vi "setCurrent.vi"(8 "error in (no error)":errorcluster, 11 "curent set":u16) -> (0 "error out":errorcluster)   [LabVIEW 2013]
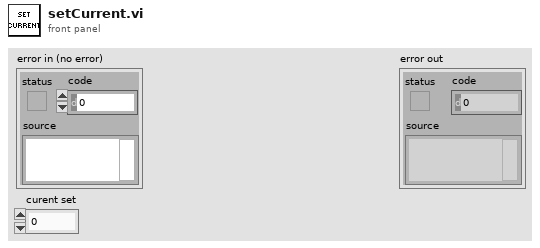
[diagram p1: front panel]
types:
  T1 = enum16{"Read", "Write", "ReadWrite", "BufferedRead", "BufferedReadWrite"}
  T2 = cluster{"data string":string, "data string":string, "data string":string, "data string":string}
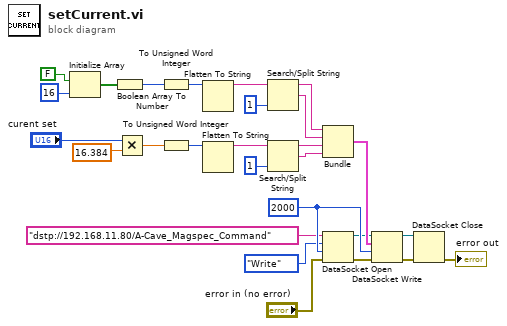
[diagram p0: block diagram]
diagram:
  w9 = 2000 ("ms timeout (10000)")
  n1 = Initialize Array(FALSE, 16 ("dimension size")) -> (w3:bool[])
  n2 = Boolean Array To Number(Boolean array=w3) -> (number=w23:u32)
  n3 = Multiply(x="curent set", y=16.384) -> (x*y=w15:dbl)
  n4 = To Unsigned Word Integer(number=w23) -> (unsigned 16bit integer=w13:u16)
  n5 = To Unsigned Word Integer(number=w15) -> (unsigned 16bit integer=w16:u16)
  n6 = Flatten To String(anything=w13) -> (data string=w19:string)  [unwired: 3 in, 2 out]
  n7 = Flatten To String(anything=w16) -> (data string=w17:string)  [unwired: 3 in, 2 out]
  n8 = Search/Split String(string=w19, offset (0)=1) -> (substring before match=w21:string, match + rest of string=w22:string)  [unwired: 1 in, 1 out]
  n9 = Search/Split String(string=w17, offset (0)=1) -> (substring before match=w10:string, match + rest of string=w11:string)  [unwired: 1 in, 1 out]
  n10 = Bundle("data string"=w21, "data string"=w22, "data string"=w10, "data string"=w11) -> (w12:T2)  [unwired: 1 in]
  n11 = DataSocket Open(8:"error in (no error)", 9:w9, 10:T1."Write" ("mode"), 11:"dstp://192.168.11.80/A-Cave_Magspec_Command" ("Target_URL")) -> (0:w8:errorcluster, 3:w6:refnum<k13>)
  n12 = DataSocket Write(8:w8, 9:w9, 10:w12, 11:w6) -> (0:w2:errorcluster, 3:w7:refnum<k13>)  [unwired: 1 out]
  n13 = DataSocket Close(8:w2, 11:w7) -> (0:→"error out":errorcluster)  [unwired: 1 in, 1 out]
